vi "2898 Teleop.vi"() -> (3 "Shooting Manual Override?":bool, 4 "Bridge Mode?":bool, 6 "Shooter Is Front":bool, 10 "Aligning Mode?":bool)   [LabVIEW 2011]
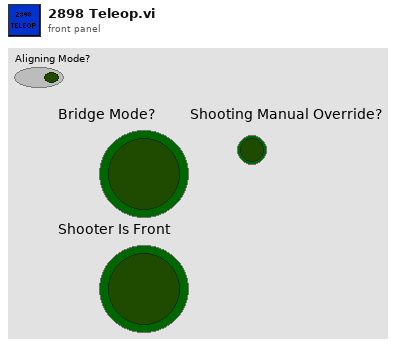
[diagram p1: front panel]
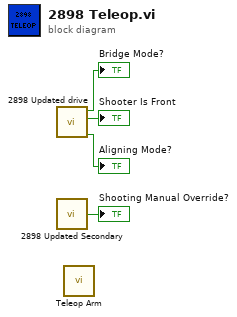
[diagram p0: block diagram]
diagram:
  n1 = call "2898 Updated drive.vi"() -> ("Aligning Mode?"=→"Aligning Mode?":bool, "Shooter is Front"=→"Shooter Is Front":bool, "Bridge Mode"=→"Bridge Mode?":bool)  [unwired: 9 in]
  n2 = call "2898 Updated Secondary.vi"() -> ("Shooting Manual Override?"=→"Shooting Manual Override?":bool)  [unwired: 15 in]
  n3 = call "Teleop Arm.vi"() -> ()  [unwired: 12 in]
